vi "624WPI_DriverStationGet Robot Mode Faster.vi"(10 "Finish":bool, 11 "DS Occurrence":refnum<k4>) -> (0 "Match Info out":T4={"Autonomous Elapsed Seconds"=0.0, "TeleOp Elapsed Seconds"=0.0, "Disabled Elapsed Seconds"=0.0, "Visited Autonomous"=FALSE, "Visited TeleOp"=FALSE, "Visited Disabled"=FALSE, "Autonomous Settings"={"Autonomous Style"=enum."Independent", "VI Refnum"=refnum}}, 1 "Control Word":T1, 2 "Call Context":T3, 3 "Robot Mode":T2)   [LabVIEW 2014]
doc: "This VI waits for control packets to arrive and determines what robot code to execute next, teletop, disable, etc. It also contains a state machine to give a first and last call context parameter and execution timings to robot code.\n\nThis software is licensed. Open the labview\\readme\\WPI Robotics Library Open Source License.txt file for more information."
uses:
  <vilib>/Rock Robotics/WPI/DriverStation/WPI_DriverStationMatch Info.ctl
  <vilib>/Rock Robotics/WPI/DriverStation/WPI_DriverStationDerivedRobotMode.ctl
  <vilib>/Rock Robotics/WPI/DriverStation/WPI_DriverStationRobotMode2.ctl
  <vilib>/Rock Robotics/SystemInterfaces/NetworkCommunication/NetComm_ControlWord.ctl
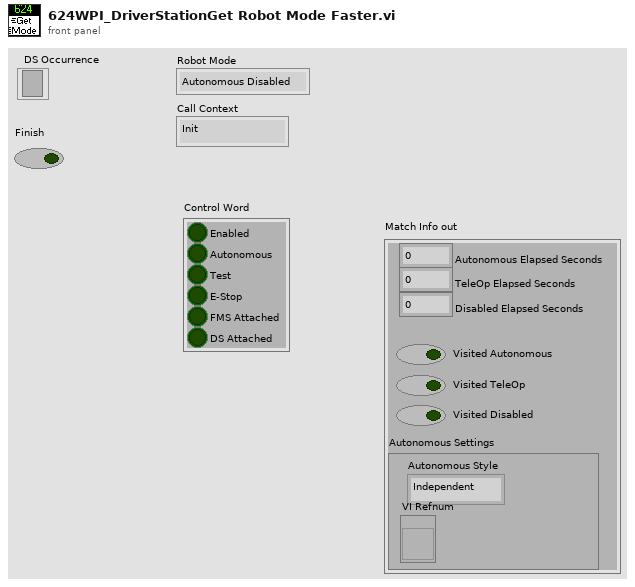
[diagram p1: front panel]
types:
  T1 = typedef "NetComm_ControlWord.ctl" = cluster{"Enabled":bool, "Autonomous":bool, "Test":bool, "E-Stop":bool, "FMS Attached":bool, "DS Attached":bool}
  T2 = typedef "WPI_DriverStationRobotMode2.ctl" = enum16{"Autonomous Disabled", "Autonomous Enabled", "Teleop Disabled", "Teleop Enabled", "Disconnected", "Finish", "Test Disabled", "Test Enabled", "Emergency Stopped"}
  T3 = typedef "WPI_DriverStationDerivedRobotMode.ctl" = enum16{"Init", "Execute", "Stop"}
  T4 = typedef "WPI_DriverStationMatch Info.ctl" = cluster{"Autonomous Elapsed Seconds":dbl, "TeleOp Elapsed Seconds":dbl, "Disabled Elapsed Seconds":dbl, "Visited Autonomous":bool, "Visited TeleOp":bool, "Visited Disabled":bool, "Autonomous Settings":cluster{"Autonomous Style":enum16{"Iterative", "Independent"}, "VI Refnum":refnum<vi>}}
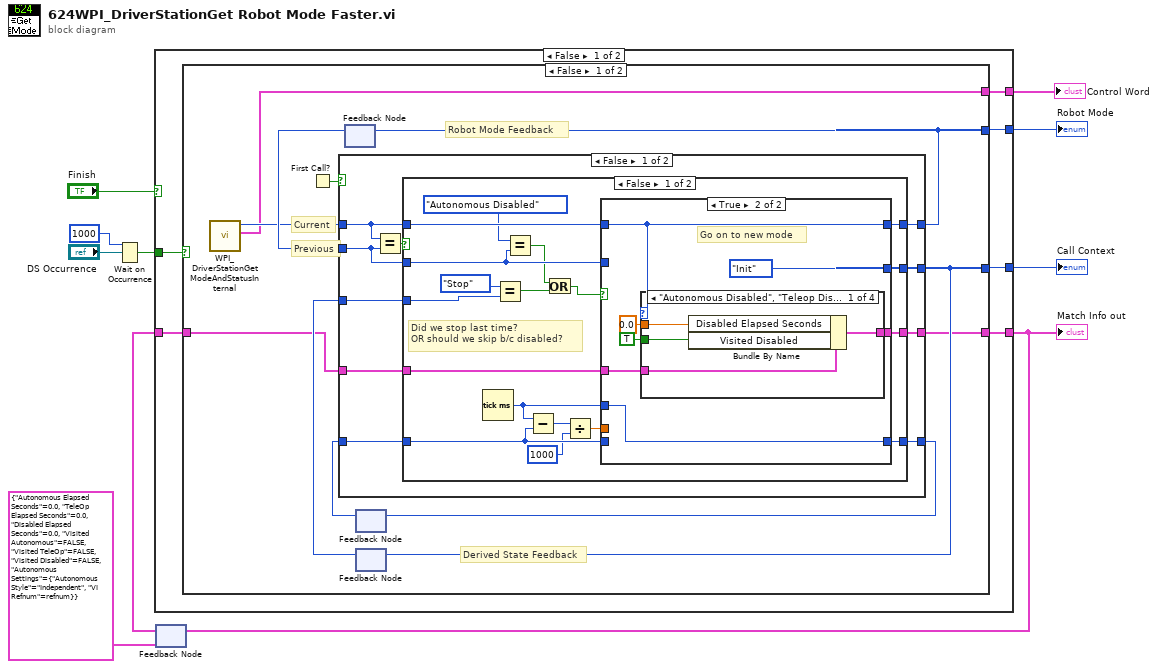
[diagram p0: block diagram]
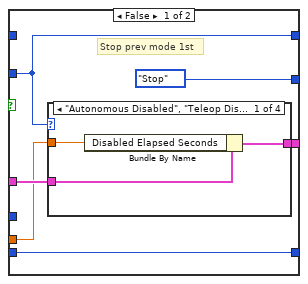
[diagram p2: hidden frame]
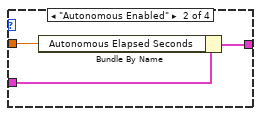
[diagram p3: hidden frame]
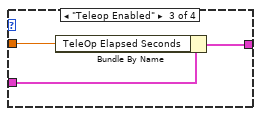
[diagram p4: hidden frame]
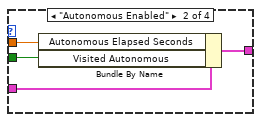
[diagram p6: hidden frame]
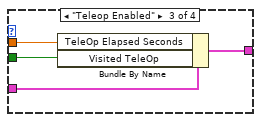
[diagram p7: hidden frame]
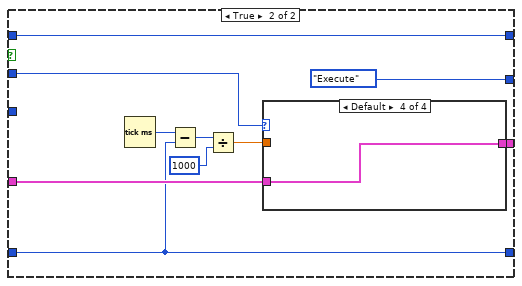
[diagram p9: hidden frame]
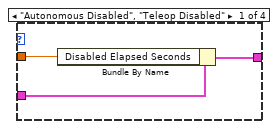
[diagram p10: hidden frame]
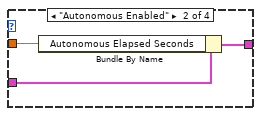
[diagram p11: hidden frame]
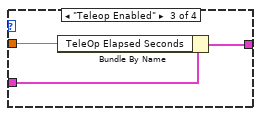
[diagram p12: hidden frame]
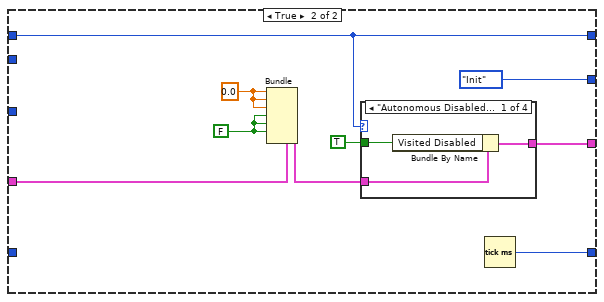
[diagram p13: hidden frame]
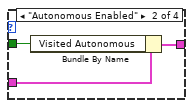
[diagram p14: hidden frame]
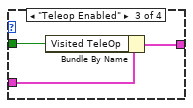
[diagram p15: hidden frame]
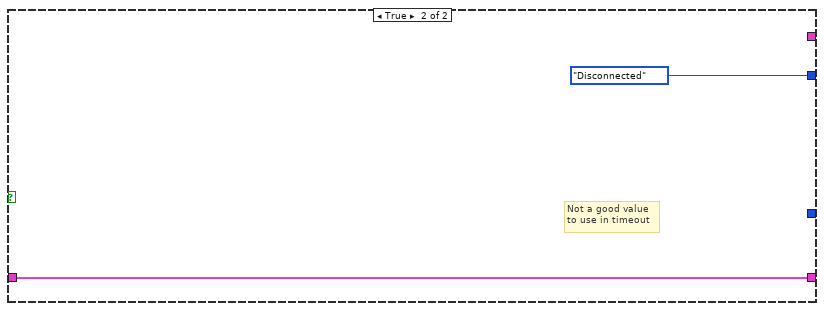
[diagram p17: hidden frame]
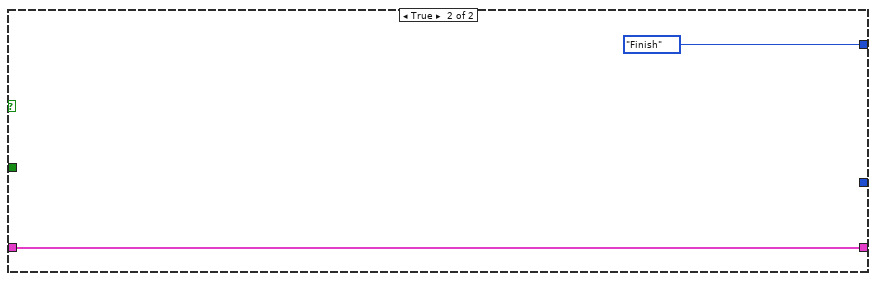
[diagram p18: hidden frame]
diagram:
  n1 = Wait on Occurrence(2:"DS Occurrence", 3:1000 ("ms timeout (-1)")) -> (0:w5:bool)  [unwired: 1 out]
  n2 = feedback #1(T4 {"Autonomous Elapsed Seconds"=0.0, "TeleOp Elapsed Seconds"=0.0, "Disabled Elapsed Seconds"=0.0, "Visited Autonomous"=FALSE, "Visited TeleOp"=FALSE, "Visited Disabled"=FALSE, "Autonomous Settings"={"Autonomous Style"=enum."Independent", "VI Refnum"=refnum}} ("Match Info")) -> (w9:T4)
  n3 = case shown="False" "Finish" {
    tunnel: [w16 _] -> w2
    tunnel: [w15 WPI_DriverStationRobotMode2."Finish" ("RobotMode")] -> w3
    tunnel: w5 -> [w14 _]
    tunnel: w9 -> [w13 w133]
    tunnel: [w12 w133] -> w8
    tunnel: [w11 _] -> w1
    frame False {
      n4 = case shown="False" w14 {
        tunnel: [w24 _] -> w16
        tunnel: [w23 WPI_DriverStationRobotMode2."Disconnected" ("RobotMode")] -> w15
        tunnel: w13 -> [w19 w131]
        tunnel: [w20 w131] -> w12
        tunnel: [w17 _] -> w11
        frame False {
          # "Derived State Feedback"
          # "Robot Mode Feedback"
          # "Previous"
          # "Current"
          n5 = call <vilib>:"WPI_DriverStationGetModeAndStatusInternal.vi"() -> ("Control Word"=w17:T1, "Robot Mode"=w18:T2)  [unwired: 10 in]
          n6 = First Call?() -> (First Call?: T/F=w25:bool)
          n7 = feedback #2() -> (w26:T2)  [unwired: 1 out]
          n8 = feedback #3() -> (w21:u32)  [unwired: 1 out]
          n9 = feedback #4() -> (w27:T3)  [unwired: 1 out]
          n10 = case shown="False" w25 {
            tunnel: [w37 w112] -> w23
            tunnel: [w36 WPI_DriverStationDerivedRobotMode."Init" ("Derived Robot State")] -> w24
            tunnel: w27 -> [w34 _]
            tunnel: w18 -> [w33 w112]
            tunnel: w26 -> [w32 _]
            tunnel: w19 -> [w31 w119]
            tunnel: [w30 w114] -> w20
            tunnel: [w28 w116] -> w22
            tunnel: w21 -> [w29 _]
            frame False {
              n11 = Equal?(x=w33, y=w32) -> (x = y?=w35:bool)
              n12 = case shown="False" w35 {
                tunnel: w33 -> [w54 w101]
                tunnel: [w53 w101] -> w37
                tunnel: [w52 WPI_DriverStationDerivedRobotMode."Execute" ("Derived Robot State")] -> w36
                tunnel: w34 -> [w55 _]
                tunnel: w32 -> [w40 w96]
                tunnel: w31 -> [w46 w97]
                tunnel: [w50 w98] -> w30
                tunnel: w29 -> [w47 w95]
                tunnel: [w48 w95] -> w28
                frame False {
                  # "Did we stop last time?\nOR should we skip b/c disabled?"
                  n13 = Tick Count (ms)() -> (millisecond timer value=w49:u32)
                  n14 = Equal?(x=WPI_DriverStationDerivedRobotMode."Stop" ("Derived Robot State"), y=w55) -> (x = y?=w42:bool)
                  n15 = Equal?(x=WPI_DriverStationRobotMode2."Autonomous Disabled", y=w40) -> (x = y?=w38:bool)
                  n16 = Subtract(x=w49, y=w47) -> (x-y=w45:u32)
                  n17 = Or(x=w38, y=w42) -> (x .or. y?=w41:bool)
                  n18 = Divide(x=w45, y=1000) -> (x/y=w44:dbl)
                  n19 = case shown="True" w41 {
                    tunnel: w54 -> [_ w77]
                    tunnel: [w56 w77] -> w53
                    tunnel: [WPI_DriverStationDerivedRobotMode."Stop" ("Derived Robot State") WPI_DriverStationDerivedRobotMode."Init" ("Derived Robot State")] -> w52
                    tunnel: w40 -> [w56 _]
                    tunnel: w46 -> [w59 w75]
                    tunnel: [w60 w74] -> w50
                    tunnel: w44 -> [w58 _]
                    tunnel: w49 -> [_ w72]
                    tunnel: [w57 w72] -> w48
                    tunnel: w47 -> [w57 _]
                    frame False {
                      # "Stop prev mode 1st"
                      n20 = case shown="\"Autonomous Disabled\", \"Teleop Disabled\"" w56 {
                        tunnel: w58 -> [w64 w67 w70 _]
                        tunnel: w59 -> [w63 w66 w69 w71]
                        tunnel: [w62 w65 w68 w71] -> w60
                        frame "Autonomous Disabled", "Teleop Disabled" {
                          n21 = Bundle By Name(cluster=w63, "Disabled Elapsed Seconds"=w64) -> (w62:T4)
                        }
                        frame "Autonomous Enabled" {
                          n22 = Bundle By Name(cluster=w66, "Autonomous Elapsed Seconds"=w67) -> (w65:T4)
                        }
                        frame "Teleop Enabled" {
                          n23 = Bundle By Name(cluster=w69, "TeleOp Elapsed Seconds"=w70) -> (w68:T4)
                        }
                        frame Default {
                        }
                      }
                    }
                    frame True {
                      # "Go on to new mode"
                      n24 = case shown="\"Autonomous Disabled\", \"Teleop Disabled\"" w77 {
                        tunnel: 0.0 -> [w82 w86 w87 _]
                        tunnel: w75 -> [w81 w85 w90 w91]
                        tunnel: [w80 w84 w89 w91] -> w74
                        tunnel: TRUE -> [w79 w83 w88 _]
                        frame "Autonomous Disabled", "Teleop Disabled" {
                          n25 = Bundle By Name(cluster=w81, "Disabled Elapsed Seconds"=w82, "Visited Disabled"=w79) -> (w80:T4)
                        }
                        frame "Autonomous Enabled" {
                          n26 = Bundle By Name(cluster=w85, "Autonomous Elapsed Seconds"=w86, "Visited Autonomous"=w83) -> (w84:T4)
                        }
                        frame "Teleop Enabled" {
                          n27 = Bundle By Name(cluster=w90, "TeleOp Elapsed Seconds"=w87, "Visited TeleOp"=w88) -> (w89:T4)
                        }
                        frame Default {
                        }
                      }
                    }
                  }
                }
                frame True {
                  n28 = Tick Count (ms)() -> (millisecond timer value=w99:u32)
                  n29 = Subtract(x=w99, y=w95) -> (x-y=w93:u32)
                  n30 = Divide(x=w93, y=u32 1000) -> (x/y=w94:dbl)
                  n31 = case shown="Default" w96 {
                    tunnel: w94 -> [w104 w107 w110 _]
                    tunnel: w97 -> [w103 w106 w109 w111]
                    tunnel: [w102 w105 w108 w111] -> w98
                    frame "Autonomous Disabled", "Teleop Disabled" {
                      n32 = Bundle By Name(cluster=w103, "Disabled Elapsed Seconds"=w104) -> (w102:T4)
                    }
                    frame "Autonomous Enabled" {
                      n33 = Bundle By Name(cluster=w106, "Autonomous Elapsed Seconds"=w107) -> (w105:T4)
                    }
                    frame "Teleop Enabled" {
                      n34 = Bundle By Name(cluster=w109, "TeleOp Elapsed Seconds"=w110) -> (w108:T4)
                    }
                    frame Default {
                    }
                  }
                }
              }
            }
            frame True {
              w118 = 0.0
              w117 = FALSE
              n35 = Bundle(cluster=w119, "Autonomous Elapsed Seconds"=w118, "TeleOp Elapsed Seconds"=w118, "Disabled Elapsed Seconds"=w118, "Visited Autonomous"=w117, "Visited TeleOp"=w117, "Visited Disabled"=w117) -> (w115:T4)  [unwired: 1 out]
              n36 = case shown="\"Autonomous Disabled\", \"Teleop Disabled\"" w112 {
                tunnel: w115 -> [w123 w126 w129 w130]
                tunnel: [w122 w125 w128 w130] -> w114
                tunnel: TRUE -> [w121 w124 w127 _]
                frame "Autonomous Disabled", "Teleop Disabled" {
                  n37 = Bundle By Name(cluster=w123, "Visited Disabled"=w121) -> (w122:T4)
                }
                frame "Autonomous Enabled" {
                  n38 = Bundle By Name(cluster=w126, "Visited Autonomous"=w124) -> (w125:T4)
                }
                frame "Teleop Enabled" {
                  n39 = Bundle By Name(cluster=w129, "Visited TeleOp"=w127) -> (w128:T4)
                }
                frame Default {
                }
              }
              n40 = Tick Count (ms)() -> (millisecond timer value=w116:u32)
            }
          }
          n41 = feedback-in #2(w23) -> ()
          n42 = feedback-in #3(w22) -> ()
          n43 = feedback-in #4(w24) -> ()
        }
        frame True {
          # "Not a good value\nto use in timeout"
        }
      }
    }
    frame True {
    }
  }
  "Robot Mode" <- w3
  "Call Context" <- w2
  "Match Info out" <- w8
  "Control Word" <- w1
  n44 = feedback-in #1(w8) -> ()
